vi "dynanometer_DAQ_analog_output.vi"() -> ()   [LabVIEW 2015]
uses:
  <vilib>/Vernier/SensorDAQ/Low Level Drivers/SensorDAQ Controls/Config Ch 1-3 Enum.ctl
  <vilib>/Vernier/SensorDAQ/Low Level Drivers/SensorDAQ Controls/Collection Parameters Enum.ctl
  <vilib>/Vernier/SensorDAQ/Low Level Drivers/SensorDAQ Controls/Config Analog Out Enum.ctl
  <vilib>/Vernier/SensorDAQ/Low Level Drivers/SensorDAQ Controls/AO Enum.ctl
  <vilib>/Utility/file.llb/Write Delimited Spreadsheet (DBL).vi
panel:
  in  "Save to File":bool=TRUE
  in  "Threshold for Ch. 2 (N)":dbl=10.0
  out "Comparison Result \n             for Ch. 2":bool[](array[boolean])
  out "Comparison Result \n           for Ch. 1":bool[](array[boolean])
  in  "Threshold for Ch. 1 (N)":dbl=10.0
  out "Ch. 2 Chart":dbl[](graph)
  out "Total # of samples":i32
  out "Time per sample \n(s/sample)":dbl
  out "AI1 Chart":dbl[](graph)
  out "AI0 Chart":dbl[](graph)
  out "Ch. 1 Chart":dbl[](graph)
  in  "?":bool
  out "SensorDAQ Connected?":bool
  in  "AI1 Configuration":T1(ring)=enum."AI1 0-5V RSE"
  in  "AI0 Configuration":T2(ring)=enum."AI0 0-5V RSE"
  in  "Repeat Collection?":bool
  in  "Samples to be Collected":dbl=20000.0
  in  "Sampling Rate (samples/s)":dbl=20.0
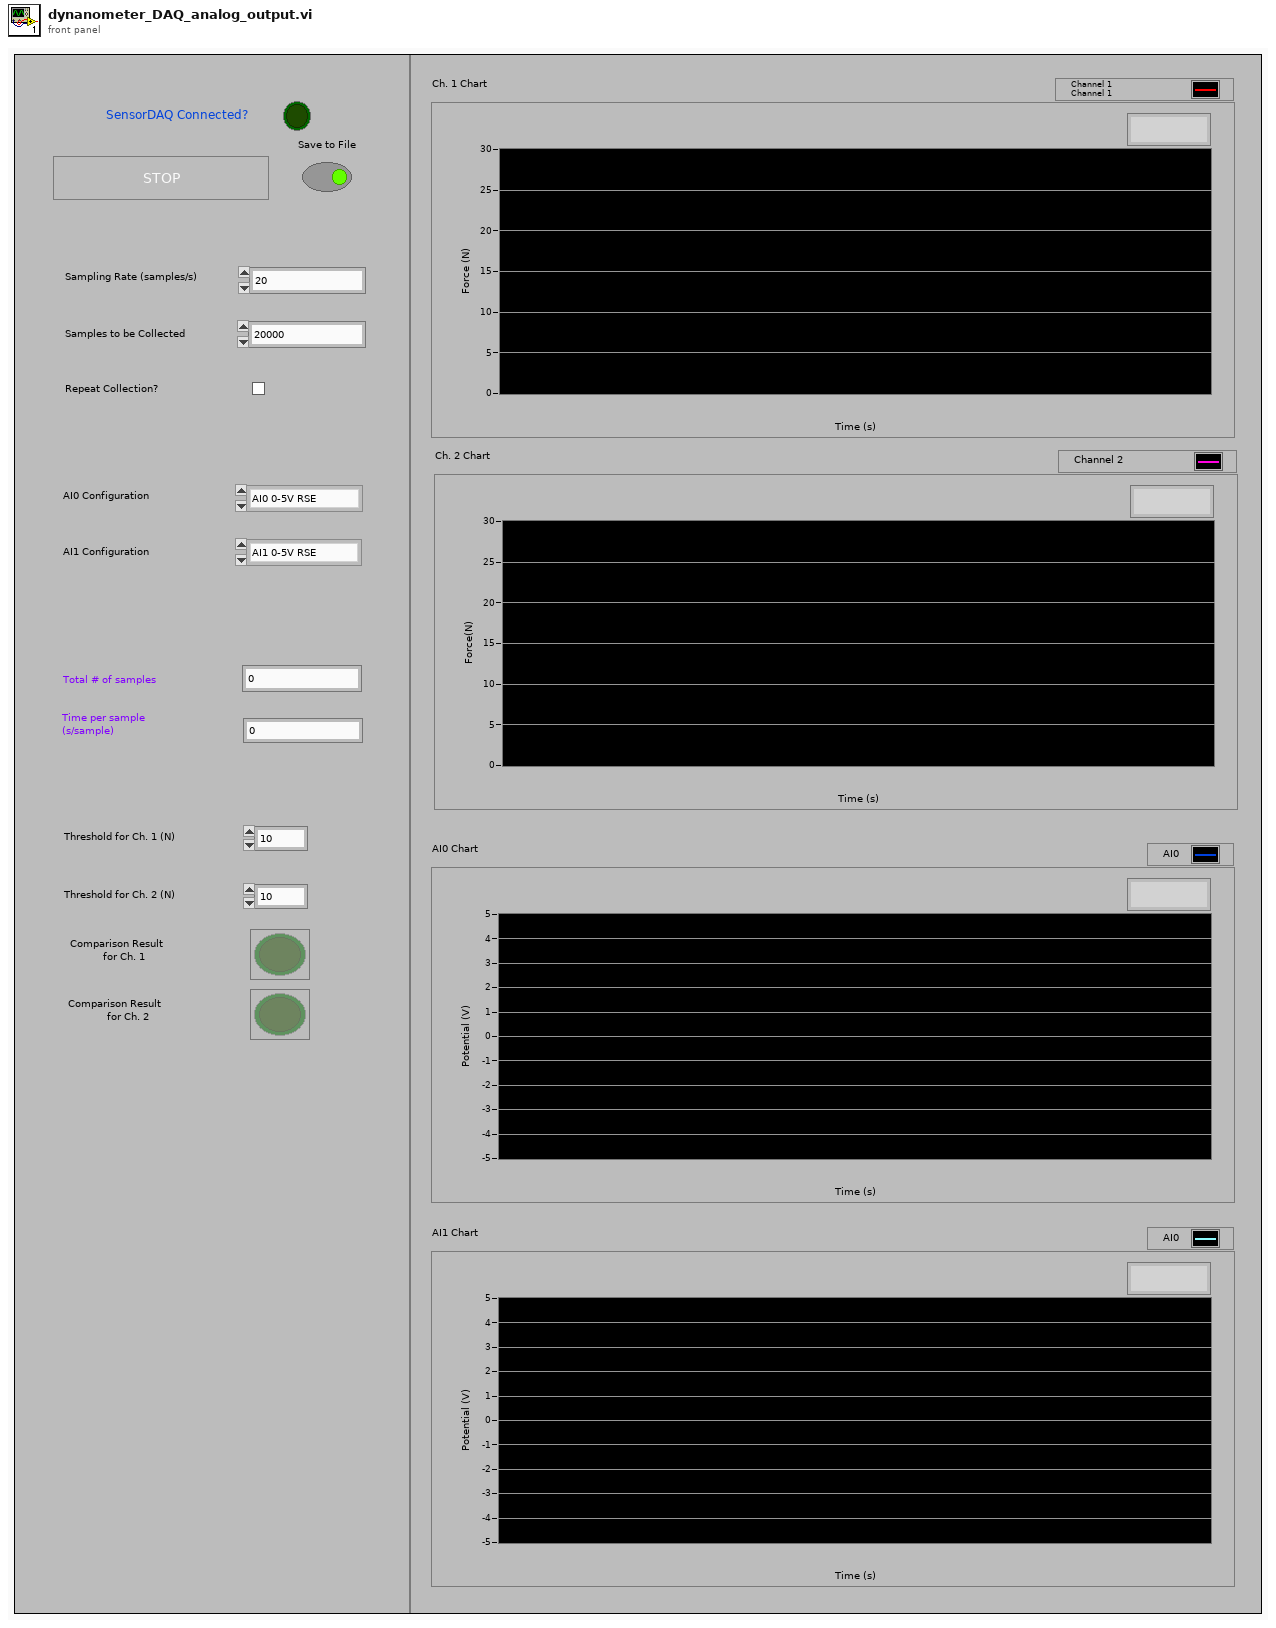
[diagram p1: front panel]
types:
  T1 = enum16{"AI1 OFF", "AI1 0-5V RSE", "AI1 +-10V RSE"}
  T2 = enum16{"AI0 OFF", "AI0 0-5V RSE", "AI0 +-10V RSE", "AI0 Differential"}
  T3 = typedef "Config Analog Out Enum.ctl" = enum16{"OFF", "ON"}
  T4 = typedef "Collection Parameters Enum.ctl" = enum16{"Modify with Inputs into this subVI", "Modify with Data Collection Popup ", "Modify with Calibration File Popup", "Modify with Select Units Popup", "Modify with Zero Reading Popup", "Get Current Parameters", "Init", "In Probe Data", "In New Parameters"}
  T5 = typedef "Config Ch 1-3 Enum.ctl" = enum16{"OFF", "ON ", "ON - Use \"Custom Ch\" Input Values"}
  T6 = typedef "DAQmx Task Cluster.ctl" = cluster{"DIG Ch Task":refnum<k21>, "P0<0:3> DigOut Task":refnum<k21>, "P0<0:3> DigIn Task":refnum<k21>, "AO 0 Task":refnum<k21>, "PFI 0 Task":refnum<k21>, "Ch1-3 AI0 AI1 Task":refnum<k21>, "SensorDAQ Device":tag}
  T7 = typedef "Setup Parameters Cluster.ctl" = cluster{"Config Ch1-3, AI0, AI1":T8, "Config DIG Ch":T12, "Config DIO":T14, "Config AO":T3, "Config Counter":T16}
  T8 = typedef "Config Ch1-3, AI0, AI1 Cluster.ctl" = cluster{"Sensor Info Array":T9[], "CH1 Y min":dbl, "CH2 Y min":dbl, "CH3 Y min":dbl, "AI0 Y min":dbl, "AI1 Y min":dbl, "CH1 Y max":dbl, "CH2 Y max":dbl, "CH3 Y max":dbl, "AI0 Y max":dbl, "AI1 Y max":dbl, "X min":dbl, "X max":dbl, "sample rate (sample/sec)":dbl, "sample time (sec/sample)":dbl, "# of samples":u32, "Repeat?":bool, "Active Channel Array":bool[], "# active probes":u32, "TrigType":T10, "TrigChan":i32, "TrigThresh":dbl, "Pre-Store (%)":i32, "Pre-store (#samp)":u32, "Short Sensor Name":string[], "Product ID Array":u8[], "AI0 Configuration":enum16{"AI0 OFF", "AI0 0-5V RSE", "AI0 +-10V RSE", "AI0 Differential"}, "AI1 Configuration":enum16{"AI1 OFF", "AI1 0-5V RSE", "AI1 +-10V RSE"}, "Averaging Enum":T11}
  T9 = typedef "Sensor Info Cluster.ctl" = cluster{"Long Name":string, "Active CalPage":u8, "Calpage Coefficients":cluster{"K0":sgl, "K1":sgl, "K2":sgl, "Units":string}[], "Equation Type":u8, "Operation Type":u8, "Num Valid Cal Pages":u8}
  T10 = typedef "TrigType Enum.ctl" = enum16{"No Trigger", "DIG Channel Trigger - Rising Edge", "DIG Channel Trigger - Falling Edge", "Screw Terminal (PFI.0) - Rising Edge", "Screw Terminal (PFI.0) - Falling Edge", "Analog Trigger - Threshold Above", "Analog Trigger - Threshold Below", "Analog Trigger - Rising", "Analog Trigger - Falling"}
  T11 = typedef "Averaging Enum.ctl" = enum16{"Averaging On", "Averaging Off"}
  T12 = typedef "Config DIG Channel Cluster.ctl" = cluster{"Config DIG Channel (OFF)":T13, "sample rate\n(sample/sec)":dbl, "# of samples":u32, "Y min":dbl, "Y max":dbl, "X min":dbl, "X max":dbl}
  T13 = typedef "Config DIG Channel Enum.ctl" = enum16{"OFF", "Photogate Simple Counting", "Photogate Single Timed Count", "Photogate Timing (Semi-Period)", "Photogate Timing (Period)", "Photogate Timing (2 Edge)", "Motion Detector", "DCU", "DCU - Pulse Train (line D1)", "Rotary Motion Sensor", "Radiation Monitor", "Heat Pulser"}
  T14 = typedef "Config DI0 Terminals Cluster.ctl" = cluster{"Dig Line P0.0":T15, "Dig Line P0.1":T15, "Dig Line P0.2":T15, "Dig Line P0.3":T15}
  T15 = typedef "Config DIO Line Enum.ctl" = enum16{"OFF", "ON - Digital In", "ON - Digital Out"}
  T16 = typedef "Config Counter Enum.ctl" = enum16{"OFF", "Simple Edge Counting", "Semi-Period Measurement", "Period Measurement", "Two Edge Separation", "Pulse Train Generation"}
  T17 = typedef "AO Enum.ctl" = enum16{"Set Output Voltage to 0 Volts", "Output Voltage on Indefinitely", "Output Voltage on for Set Time"}
  T18 = typedef "NI_Matrix.lvlib/RealMatrix.ctl" = dbl[][]
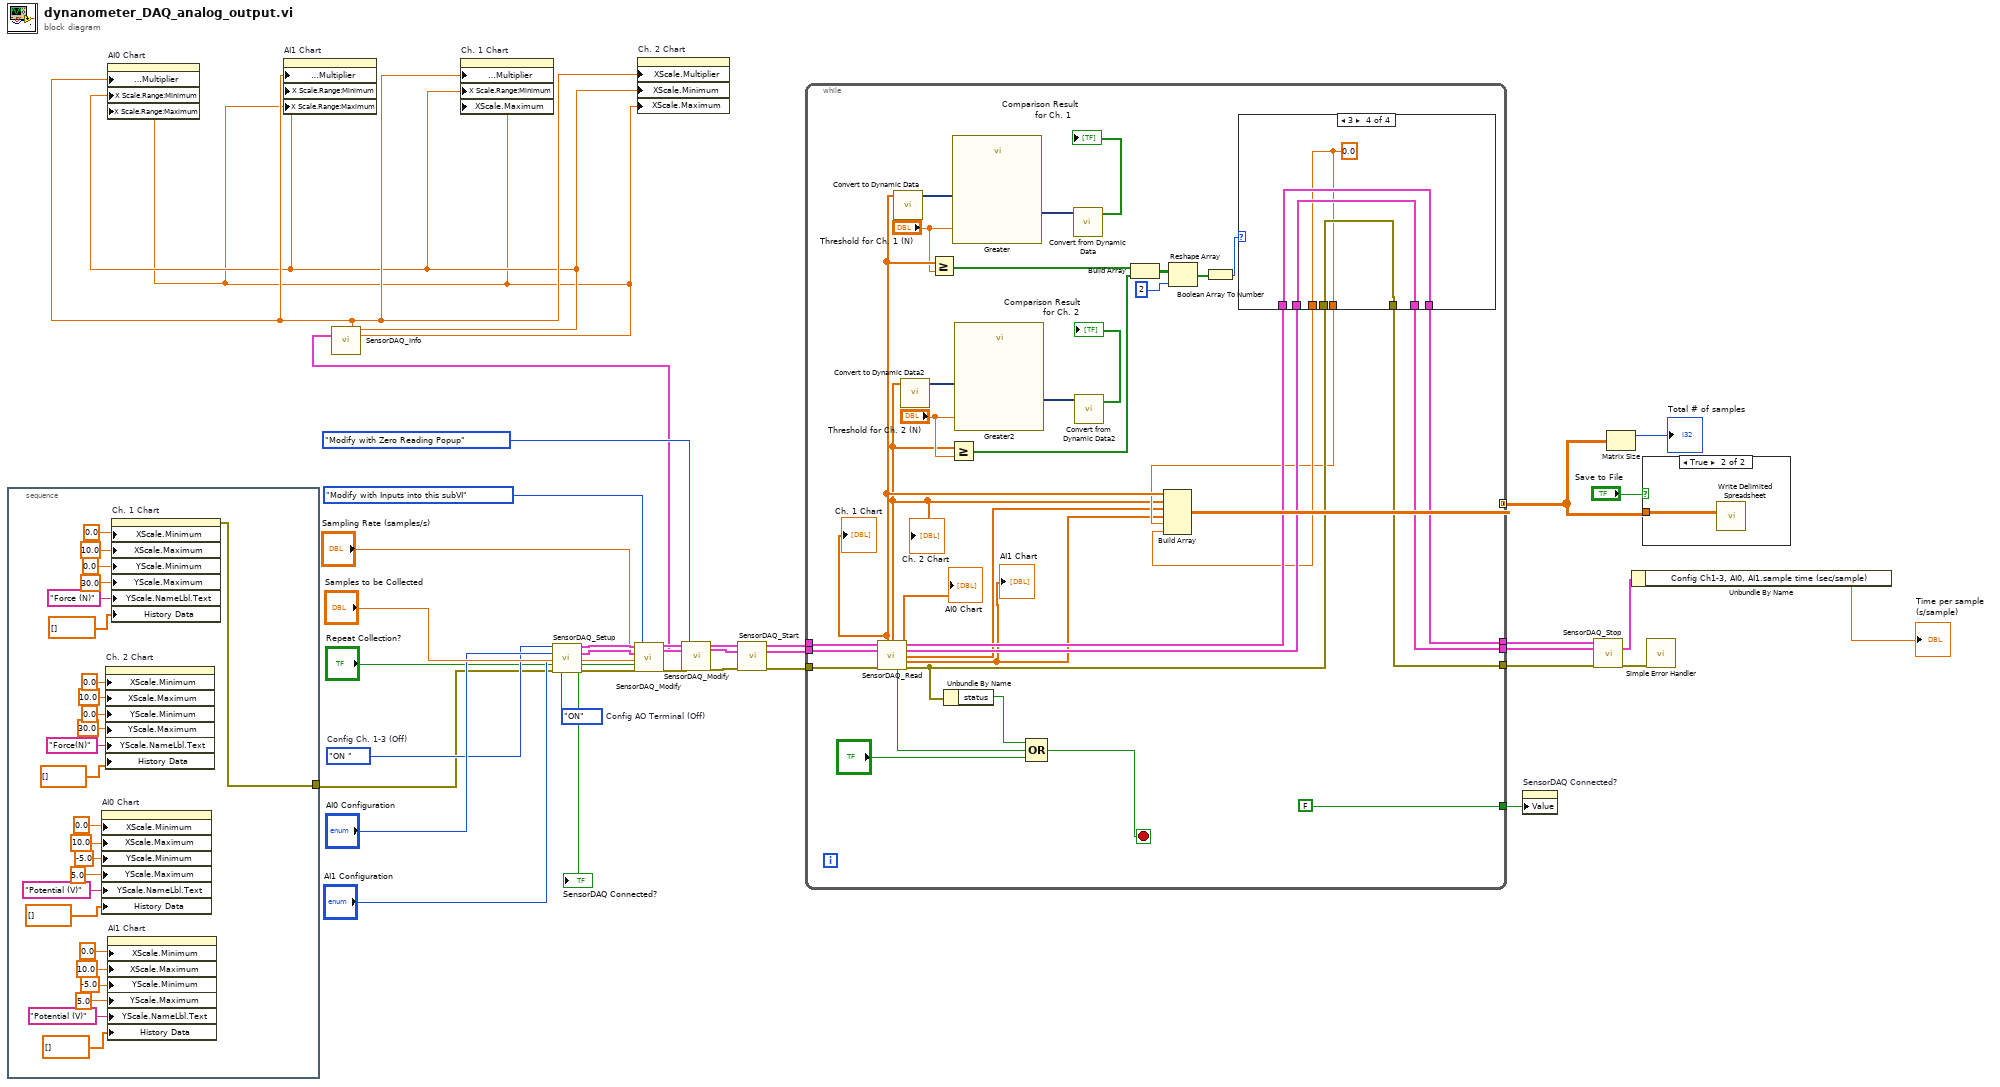
[diagram p0: block diagram]
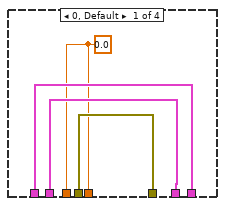
[diagram p3: hidden frame]
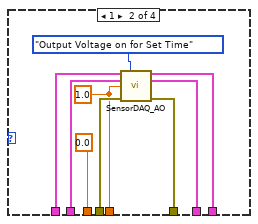
[diagram p4: hidden frame]
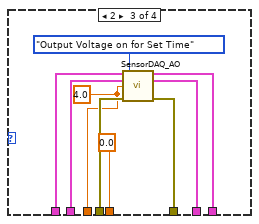
[diagram p5: hidden frame]
diagram:
  w9 = Config_Analog_Out_Enum."ON"  # Config AO Terminal (Off)
  w32 = Config_Ch_1-3_Enum."ON "  # Config Ch. 1-3 (Off)
  n1 = stacked-sequence {
    tunnel: [w43] -> w15
    frame #0 {
      n2 = property on="AI0 Chart" class="WFChart (strict)"("XScale.Minimum"=0.0, "XScale.Maximum"=10.0, "YScale.Minimum"=-5.0, "YScale.Maximum"=5.0, "YScale.NameLbl.Text"="Potential (V)", "History Data"=dbl[] [] ("Ch. 1 Graph")) -> ()  [unwired: 2 in, 2 out]
      n3 = property on="Ch. 2 Chart" class="WFChart (strict)"("XScale.Minimum"=0.0 ("X Scale.Range:Minimum"), "XScale.Maximum"=10.0 ("X Scale.Range:Maximum"), "YScale.Minimum"=0.0 ("Y Scale.Range:Minimum"), "YScale.Maximum"=30.0 ("Y Scale.Range:Maximum"), "YScale.NameLbl.Text"="Force(N)" ("Y Scale.Name Label.Text"), "History Data"=dbl[] []) -> ()  [unwired: 2 in, 2 out]
      n4 = property on="AI1 Chart" class="WFChart (strict)"("XScale.Minimum"=0.0, "XScale.Maximum"=10.0, "YScale.Minimum"=-5.0, "YScale.Maximum"=5.0, "YScale.NameLbl.Text"="Potential (V)", "History Data"=dbl[] [] ("Ch. 1 Graph")) -> ()  [unwired: 2 in, 2 out]
      n5 = property on="Ch. 1 Chart" class="WFChart (strict)"("XScale.Minimum"=0.0, "XScale.Maximum"=10.0, "YScale.Minimum"=0.0, "YScale.Maximum"=30.0, "YScale.NameLbl.Text"="Force (N)", "History Data"=dbl[] [] ("Ch. 1 Graph")) -> (error out=w43:errorcluster)  [unwired: 2 in, 1 out]
    }
  }
  n6 = call <vilib>:"SensorDAQ_Setup.vi"("Config Ch. 1-3 (Off)"=w32, "AI0 Configuration (Off)"="AI0 Configuration", "AI1 Configuration (Off)"="AI1 Configuration", "error in (no error)"=w15, "Config AO Terminal (Off)"=w9) -> ("DAQmx Task Cluster"=w36:T6, "Setup Parameters"=w35:T7, "SensorDAQ Connected?"=→"SensorDAQ Connected?":bool, "Error Out"=w28:errorcluster)  [unwired: 7 in]
  n7 = call <vilib>:"SensorDAQ_Modify.vi"("DAQmx Task Cluster"=w36, "Setup Parameters"=w35, "Sample Rate (samples/sec)"="Sampling Rate (samples/s)", "Samples to be Collected"="Samples to be Collected", "Repeat Collection?"="Repeat Collection?", "error in (no error)"=w28, "Collection Parameters Enum"=Collection_Parameters_Enum."Modify with Inputs into this subVI") -> ("DAQmx Task Cluster out"=w25:T6, "Setup Parameters"=w24:T7, "error out"=w20:errorcluster)  [unwired: 8 in, 2 out]
  n8 = call <vilib>:"SensorDAQ_Modify.vi"("DAQmx Task Cluster"=w25, "Setup Parameters"=w24, "error in (no error)"=w20, "Collection Parameters Enum"=Collection_Parameters_Enum."Modify with Zero Reading Popup") -> ("DAQmx Task Cluster out"=w21:T6, "Setup Parameters"=w10:T7, "error out"=w19:errorcluster)  [unwired: 11 in, 2 out]
  n9 = call <vilib>:"SensorDAQ_Info.vi"("Setup Parameters"=w10) -> ("X Multiplier"=w14:dbl, "X min"=w13:dbl, "X max"=w12:dbl)  [unwired: 7 in, 5 out]
  n10 = property on="AI0 Chart" class="WFChart (strict)"("X Scale.Offset and Multiplier:Multiplier"=w14, "X Scale.Range:Minimum"=w13, "X Scale.Range:Maximum"=w12) -> ()  [unwired: 2 in, 2 out]
  n11 = property on="AI1 Chart" class="WFChart (strict)"("X Scale.Offset and Multiplier:Multiplier"=w14, "X Scale.Range:Minimum"=w13, "X Scale.Range:Maximum"=w12) -> ()  [unwired: 2 in, 2 out]
  n12 = property on="Ch. 1 Chart" class="WFChart (strict)"("X Scale.Offset and Multiplier:Multiplier"=w14, "X Scale.Range:Minimum"=w13, "XScale.Maximum"=w12) -> ()  [unwired: 2 in, 2 out]
  n13 = property on="Ch. 2 Chart" class="WFChart (strict)"("XScale.Multiplier"=w14, "XScale.Minimum"=w13, "XScale.Maximum"=w12) -> ()  [unwired: 2 in, 2 out]
  n14 = call <vilib>:"SensorDAQ_Start.vi"("DAQmx Task Cluster"=w21, "Setup Parameters"=w10, "error in"=w19) -> ("DAQmx Task Cluster out"=w8:T6, "Setup Parameters"=w7:T7, "error out"=w6:errorcluster)  [unwired: 10 in]
  n15 = while {
    tunnel: w8 -> [w90]
    tunnel: w7 -> [w89]
    tunnel: w6 -> [w91]
    tunnel: [FALSE] -> w27
    tunnel: [w92] -> w2 mode=concatenating
    tunnel: [w74] -> w5
    tunnel: [w75] -> w4
    tunnel: [w76] -> w3
    stop <- w96 stop-if-true
    n16 = call <vilib>:"SensorDAQ_Read.vi"("DAQmx Task Cluster"=w90, "Setup Parameters"=w89, "error in"=w91) -> ("CH 1"=w72:dbl[], "CH 2"=w64:dbl[], "DAQmx Task Cluster"=w79:T6, "Setup Parameters"=w78:T7, "AI0"=w63:dbl[], "AI1"=w62:dbl[], "Collection Done"=w94:bool, "error out"=w77:errorcluster)  [unwired: 2 in, 3 out]
    "Ch. 1 Chart" <- w72
    "AI0 Chart" <- w63
    "AI1 Chart" <- w62
    "Ch. 2 Chart" <- w64
    n17 = call "Convert to Dynamic Data"("Array"=w72) -> ("Dynamic Data Type"=w88:dynamicdata)  [unwired: 3 in]
    n18 = call "Convert to Dynamic Data2"("Array"=w64) -> ("Dynamic Data Type"=w86:dynamicdata)  [unwired: 3 in]
    n19 = Greater Or Equal?(x=w72, y="Threshold for Ch. 1 (N)") -> (x >= y?=w70:bool[])
    n20 = Unbundle By Name(w77) -> ("status"=w95:bool)
    n21 = Greater Or Equal?(x=w64, y="Threshold for Ch. 2 (N)") -> (x >= y?=w68:bool[])
    n22 = call "Greater"("Operand 2"="Threshold for Ch. 1 (N)", "Operand 1"=w88) -> ("Result"=w73:dynamicdata)  [unwired: 8 in, 1 out]
    n23 = call "Greater2"("Operand 2"="Threshold for Ch. 2 (N)", "Operand 1"=w86) -> ("Result"=w87:dynamicdata)  [unwired: 8 in, 1 out]
    n24 = Compound Arithmetic op=OR(w95, w94, "?") -> (w96:bool)
    n25 = call "Convert from Dynamic Data"("Dynamic Data Type"=w73) -> ("Array"=→"Comparison Result \n           for Ch. 1":bool[])  [unwired: 3 in]
    n26 = call "Convert from Dynamic Data2"("Dynamic Data Type"=w87) -> ("Array"=→"Comparison Result \n             for Ch. 2":bool[])  [unwired: 3 in]
    n27 = Build Array(w70, w68) -> (w82:bool[][])
    n28 = Reshape Array(w82, 2 ("dimension size")) -> (w67:bool[])
    n29 = Boolean Array To Number(Boolean array=w67) -> (number=w80:u32)
    n30 = case shown="3" w80 {
      tunnel: w79 -> [w100 w108 w117 w122]
      tunnel: w78 -> [w99 w107 w116 w121]
      tunnel: w77 -> [w98 w106 w115 w120]
      tunnel: [w98 w105 w114 w120] -> w76
      tunnel: [w99 w104 w113 w121] -> w75
      tunnel: [w100 w103 w112 w122] -> w74
      tunnel: [w97 0.0 w111 w119] -> w66
      tunnel: [w97 w102 0.0 w119] -> w65
      frame 0, Default {
        w97 = 0.0
      }
      frame 1 {
        w102 = 1.0 ("Output Voltage")
        n31 = call <vilib>:"SensorDAQ_AO.vi"("DAQmx Task Cluster"=w108, "AO Setup"=AO_Enum."Output Voltage on for Set Time", "Setup Parameters"=w107, "Output Voltage"=w102, "error in (no error)"=w106) -> ("DAQmx Task Cluster"=w103:T6, "Setup Parameters"=w104:T7, "error out"=w105:errorcluster)  [unwired: 8 in]
      }
      frame 2 {
        w111 = 4.0 ("Output Voltage")
        n32 = call <vilib>:"SensorDAQ_AO.vi"("DAQmx Task Cluster"=w117, "AO Setup"=AO_Enum."Output Voltage on for Set Time", "Setup Parameters"=w116, "Output Voltage"=w111, "error in (no error)"=w115) -> ("DAQmx Task Cluster"=w112:T6, "Setup Parameters"=w113:T7, "error out"=w114:errorcluster)  [unwired: 8 in]
      }
      frame 3 {
        w119 = 0.0
      }
    }
    n33 = Build Array(w72, w64, w63, w62, w65, w66) -> (w92:T18)
  }
  n34 = property on="SensorDAQ Connected?" class="Bool (strict)"("Value"=w27) -> ()  [unwired: 2 in, 2 out]
  n35 = call <vilib>:"SensorDAQ_Stop.vi"("DAQmx Task Cluster"=w5, "Setup Parameters"=w4, "error in"=w3) -> ("Setup Parameters"=w18:T7, "error out"=w11:errorcluster)  [unwired: 10 in, 1 out]
  n36 = Matrix Size(0:w2) -> (1:→"Total # of samples":i32)  [unwired: 1 out]
  n37 = Unbundle By Name(w18) -> ("Config Ch1-3, AI0, AI1.sample time (sec/sample)"=→"Time per sample \n(s/sample)":dbl)
  n38 = case shown="True" "Save to File" {
    tunnel: w2 -> [_ w123]
    frame False {
    }
    frame True {
      n39 = call-poly <vilib>:"Write Delimited Spreadsheet.vi"("2D data"=w123) -> ()  [unwired: 13 in, 2 out]
    }
  }
  n40 = call <vilib>:"Simple Error Handler.vi"("error in (no error)"=w11) -> ()  [unwired: 4 in, 5 out]
